vi "Time.DateTime Adjust.vi"(7 "OffsetHrs":dbl, 10 "Action":T1, 11 "Time Stamp":timestamp) -> (2 "OffsetHrs Out":dbl, 3 "Time Stamp Out":timestamp)   [LabVIEW 2024]
uses:
  Time.DateTime Adjust Action.ctl
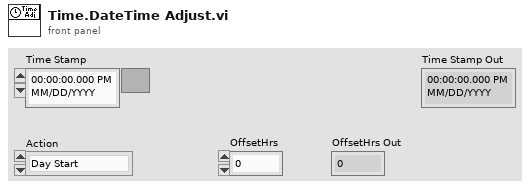
[diagram p1: front panel]
types:
  T1 = typedef "Time.DateTime Adjust Action.ctl" = enum16{"Day Start", "Day End", "Offset Hrs", "UTC to Local", "Local to UTC"}
  T2 = typedef "LVDateTimeRec.ctl" = cluster{"fractional second":dbl, "second":i32, "minute":i32, "hour":i32, "day of month":i32, "month":i32, "year":i32, "day of week":i32, "day of year":i32, "DST":i32}
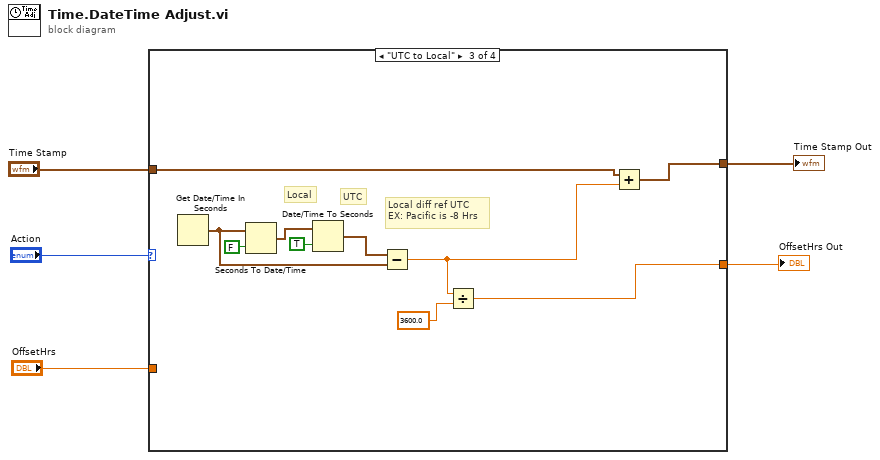
[diagram p0: block diagram]
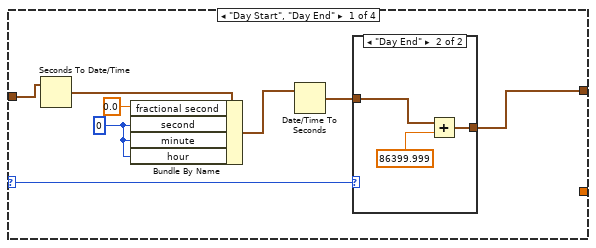
[diagram p2: hidden frame]
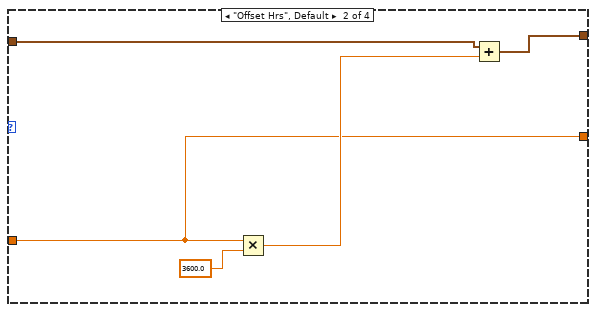
[diagram p4: hidden frame]
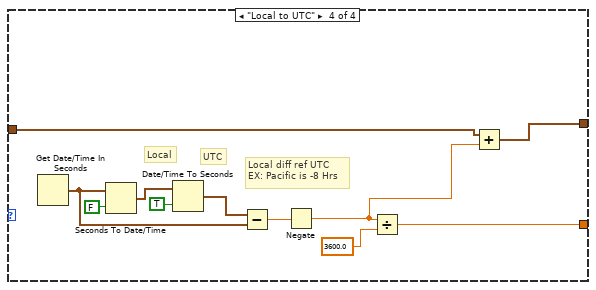
[diagram p5: hidden frame]
diagram:
  n1 = case shown="\"UTC to Local\"" "Action" {
    selector: "Action" -> [w7 _ _ _]
    tunnel: "Time Stamp" -> [w10 w22 w32 w43]
    tunnel: [w6 w21 w31 w42] -> w3
    tunnel: "OffsetHrs" -> [_ w18 _ _]
    tunnel: [_ w18 w24 w35] -> w1
    frame "Day Start", "Day End" {
      w11 = 0 ("second")
      n2 = Seconds To Date/Time(time stamp (now)=w10) -> (date time rec=w13:T2)  [unwired: 1 in]
      n3 = Bundle By Name(cluster=w13, "fractional second"=0.0, "second"=w11, "minute"=w11, "hour"=w11) -> (w9:T2)
      n4 = Date/Time To Seconds(2:w9) -> (0:w8:timestamp)  [unwired: 1 in]
      n5 = case shown="\"Day End\"" w7 {
        tunnel: w8 -> [w14 w17]
        tunnel: [w14 w15] -> w6
        frame "Day Start", Default {
        }
        frame "Day End" {
          n6 = Add(x=w17, y=86399.999) -> (x+y=w15:timestamp)
        }
      }
    }
    frame "Offset Hrs", Default {
      n7 = Multiply(x=w18, y=3600.0) -> (x*y=w19:dbl)
      n8 = Add(x=w22, y=w19) -> (x+y=w21:timestamp)
    }
    frame "UTC to Local" {
      # "Local diff ref UTC\nEX: Pacific is -8 Hrs"
      # "UTC"
      # "Local"
      n9 = Get Date/Time In Seconds() -> (seconds since 1Jan1904=w25:timestamp)
      n10 = Seconds To Date/Time(time stamp (now)=w25, to UTC (F)=FALSE) -> (date time rec=w30:T2)
      n11 = Date/Time To Seconds(1:TRUE ("to UTC (F)"), 2:w30) -> (0:w28:timestamp)
      n12 = Subtract(x=w28, y=w25) -> (x-y=w23:dbl)
      n13 = Divide(x=w23, y=3600.0) -> (x/y=w24:dbl)
      n14 = Add(x=w32, y=w23) -> (x+y=w31:timestamp)
    }
    frame "Local to UTC" {
      # "Local diff ref UTC\nEX: Pacific is -8 Hrs"
      # "UTC"
      # "Local"
      n15 = Get Date/Time In Seconds() -> (seconds since 1Jan1904=w36:timestamp)
      n16 = Seconds To Date/Time(time stamp (now)=w36, to UTC (F)=FALSE) -> (date time rec=w41:T2)
      n17 = Date/Time To Seconds(1:TRUE ("to UTC (F)"), 2:w41) -> (0:w39:timestamp)
      n18 = Subtract(x=w39, y=w36) -> (x-y=w34:dbl)
      n19 = Negate(x=w34) -> (-x=w33:dbl)
      n20 = Divide(x=w33, y=3600.0) -> (x/y=w35:dbl)
      n21 = Add(x=w43, y=w33) -> (x+y=w42:timestamp)
    }
  }
  "Time Stamp Out" <- w3
  "OffsetHrs Out" <- w1
